vi "Location to Insecure Address.vi"(11 "Location":T1) -> (3 "Address":string)   [LabVIEW 2020, in "gRPC Utilities.lvlib"]
uses:
  gRPC Utilities.lvlib
  MeasurementLink Discovery Client/RPC Messages/ni_measurementlink_discovery_v1_ServiceLocation.ctl
  MeasurementLink Discovery Client/MeasurementLink Discovery Client.lvlib
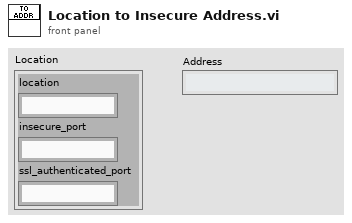
[diagram p1: front panel]
types:
  T1 = typedef "MeasurementLink Discovery Client.lvlib/ni_measurementlink_discovery_v1_ServiceLocation.ctl" = cluster{"location":string, "insecure_port":string, "ssl_authenticated_port":string}
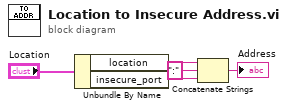
[diagram p0: block diagram]
diagram:
  n1 = Unbundle By Name("Location") -> ("location"=w5:string, "insecure_port"=w4:string)
  n2 = Concatenate Strings(w5, ":" ("string"), w4) -> (→"Address":string)
